vi "DAQ- Steper.vi"(0 "Travel (Degree)":dbl=100.0, 1 "Mode":i32(ring)=10178 items=["Finite Samples"=10178, "Continuous Samples"=10123, "Hardware Timed Single Point"=12522], 5 "Home Condition":bool, 7 "Speed d/s":dbl=10.0, 11 "error in":errorcluster) -> (4 "Task Done Bit":bool, 14 "error out":errorcluster)   [LabVIEW 2020]
uses:
  Project Setup/Globle Variable/GR_Servo.vi
  Galobal variable_TI.vi
  <vilib>/DAQmx/create/channels.llb/DAQmx Create Channel (CO-Pulse Generation-Frequency).vi
  <vilib>/DAQmx/configure/timing.llb/DAQmx Timing (Implicit).vi
panel:
  in  "Motor PPR":dbl=3600.0
  in  "Motor Gear Ratio":dbl=1.0
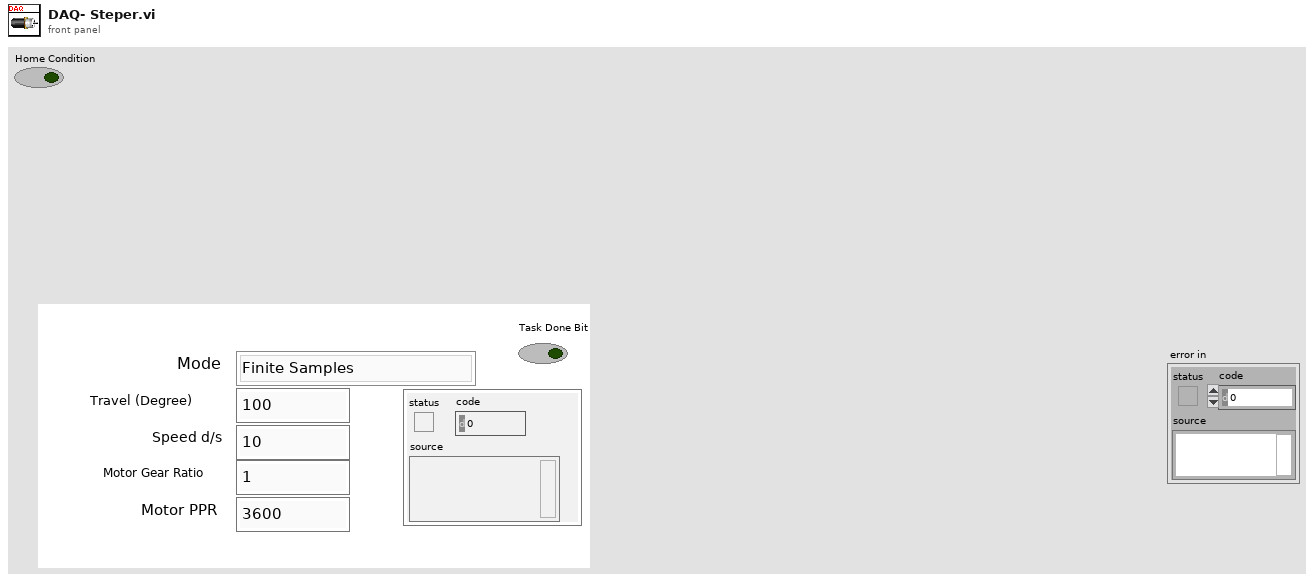
[diagram p1: front panel]
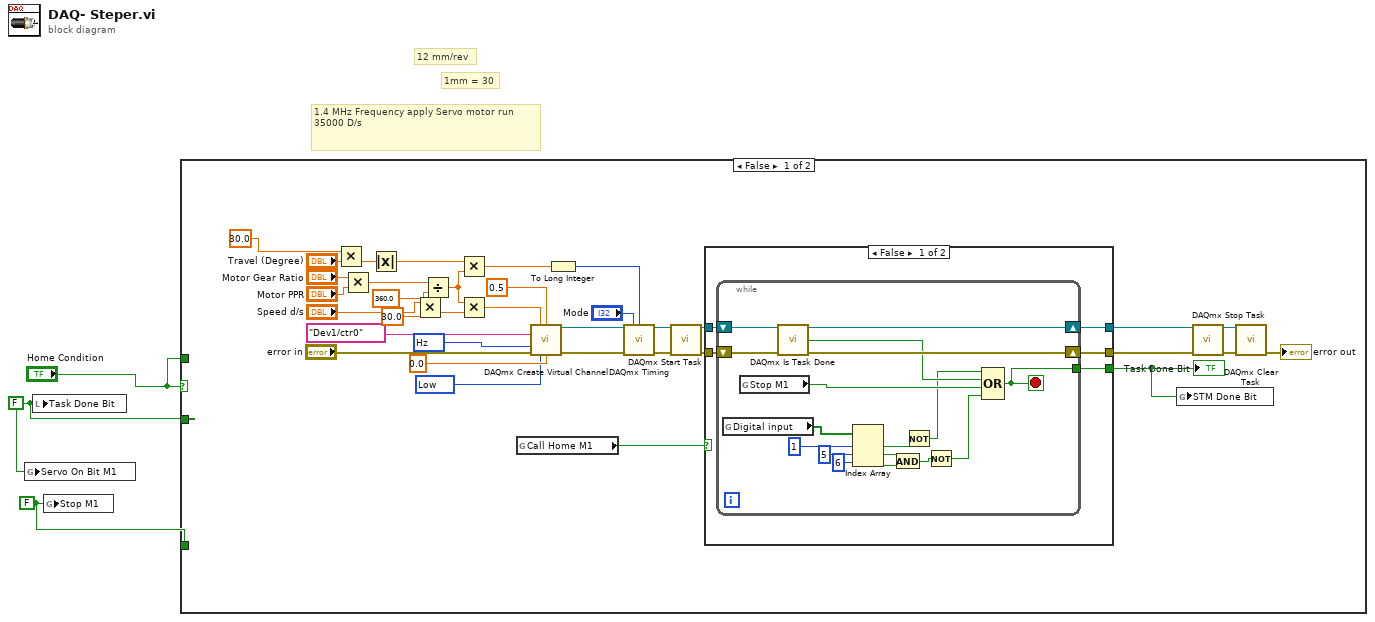
[diagram p0: block diagram]
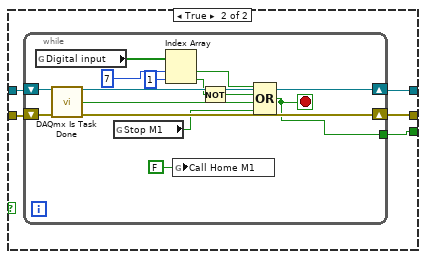
[diagram p2: hidden frame]
diagram:
  w2 = FALSE ("Stop M1")
  w3 = FALSE ("Task Done Bit")
  # "1mm = 30"
  # "12 mm/rev"
  # "1.4 MHz Frequency apply Servo motor run \n35000 D/s"
  n1 = global write "GR_Servo.vi" "Servo On Bit M1"(w3) -> ()
  n2 = local write "Task Done Bit"(w3) -> ()
  n3 = global write "Galobal variable_TI.vi" "Stop M1"(w2) -> ()
  n4 = case shown="False" "Home Condition" {
    tunnel: w3 -> [_ _]
    tunnel: w2 -> [_ _]
    tunnel: "Home Condition" -> [_ _]
    frame False {
      w14 = 10373 items=["Hz"=10373] ("units")
      w15 = 10214 items=["High"=10192, "Low"=10214] ("idle state")
      n5 = Multiply(x=30.0, y="Travel (Degree)") -> (x*y=w10:dbl)
      n6 = Multiply(x="Motor Gear Ratio", y="Motor PPR") -> (x*y=w24:dbl)
      n7 = Absolute Value(x=w10) -> (abs(x)=w23:dbl)
      n8 = Multiply(x="Speed d/s", y=30.0) -> (x*y=w8:dbl)
      n9 = Divide(x=w24, y=360.0) -> (x/y=w30:dbl)
      n10 = Multiply(x=w23, y=w30) -> (x*y=w28:dbl)
      n11 = Multiply(x=w30, y=w8) -> (x*y=w35:dbl)
      n12 = global read "Galobal variable_TI.vi" "Call Home M1"() -> (w5:bool)
      n13 = call-poly <vilib>:"DAQmx Create Virtual Channel.vi"("frequency"=w35, "duty cycle"=0.5, "counter"=tag "Dev1/ctr0", "units"=w14, "error in"="error in", "idle state"=w15, "initial delay"=0.0) -> ("task out"=w17:refnum<k21>, "error out"=w18:errorcluster)  [unwired: 7 in]
      n14 = To Long Integer(number=w28) -> (32bit integer=w38:i32)
      n15 = call-poly <vilib>:"DAQmx Timing.vi"("task/channels in"=w17, "sample mode"="Mode", "samples per channel"=w38, "error in"=w18) -> ("task out"=w19:refnum<k21>, "error out"=w20:errorcluster)  [unwired: 10 in]
      n16 = call <vilib>:"DAQmx Start Task.vi"("task/channels in"=w19, "error in"=w20) -> ("task out"=w13:refnum<k21>, "error out"=w11:errorcluster)  [unwired: 12 in]
      n17 = case shown="False" w5 {
        tunnel: [w43 w62] -> w33
        tunnel: w13 -> [w42 w65]
        tunnel: [w41 w63] -> w12
        tunnel: w11 -> [w40 w64]
        tunnel: [w39 w61] -> w4
        frame False {
          n18 = while {
            shift-right: [w58] -> w41
            shift-left: w42 -> [w60]
            shift-right: [w59] -> w43
            shift-left: w40 -> [w57]
            tunnel: [w56] -> w39
            stop <- w56 stop-if-true
            n19 = global read "Galobal variable_TI.vi" "Digital input"() -> (w55:bool[])
            n20 = global read "Galobal variable_TI.vi" "Stop M1"() -> (w53:bool)
            n21 = call <vilib>:"DAQmx Is Task Done.vi"("task/channels in"=w60, "error in"=w57) -> ("task out"=w58:refnum<k21>, "task done?"=w52:bool, "error out"=w59:errorcluster)  [unwired: 11 in]
            n22 = Index Array(array=w55, index #1=1 ("index"), index #2=5 ("index"), index #3=6 ("index")) -> (element #1=w51:bool, element #2=w47:bool, element #3=w46:bool)
            n23 = And(x=w47, y=w46) -> (x .and. y?=w45:bool)
            n24 = Not(x=w51) -> (.not. x?=w50:bool)
            n25 = Not(x=w45) -> (.not. x?=w44:bool)
            n26 = Compound Arithmetic op=OR(w50, w52, w53, w44) -> (w56:bool)
          }
        }
        frame True {
          n27 = while {
            shift-right: [w77] -> w63
            shift-left: w65 -> [w79]
            shift-right: [w78] -> w62
            shift-left: w64 -> [w76]
            tunnel: [w71] -> w61
            stop <- w71 stop-if-true
            n28 = global read "Galobal variable_TI.vi" "Digital input"() -> (w72:bool[])
            n29 = call <vilib>:"DAQmx Is Task Done.vi"("task/channels in"=w79, "error in"=w76) -> ("task out"=w77:refnum<k21>, "task done?"=w75:bool, "error out"=w78:errorcluster)  [unwired: 11 in]
            n30 = global read "Galobal variable_TI.vi" "Stop M1"() -> (w74:bool)
            n31 = Index Array(array=w72, index #1=7 ("index"), index #2=1 ("index")) -> (element #1=w67:bool, element #2=w68:bool)
            n32 = global write "Galobal variable_TI.vi" "Call Home M1"(FALSE ("Call Home M1")) -> ()
            n33 = Not(x=w68) -> (.not. x?=w66:bool)
            n34 = Compound Arithmetic op=OR(w67, w66, w75, w74) -> (w71:bool)
          }
        }
      }
      "Task Done Bit" <- w4
      n35 = global write "Galobal variable_TI.vi" "STM Done Bit"(w4) -> ()
      n36 = call <vilib>:"DAQmx Stop Task.vi"("task/channels in"=w12, "error in"=w33) -> ("task out"=w21:refnum<k21>, "error out"=w34:errorcluster)  [unwired: 12 in]
      n37 = call <vilib>:"DAQmx Clear Task.vi"("task in"=w21, "error in"=w34) -> ("error out"=→"error out":errorcluster)  [unwired: 13 in]
    }
    frame True {
    }
  }
